vi "get_all_refr_pol_corrections.vi"(8 "Error In":errorcluster, 10 "Sample":string, 11 "File Path":path) -> (0 "Error Out":errorcluster)   [LabVIEW 2019]
panel:
  out "Progress":u8(slide) scale=0.0..100.0
  # "Refration and Polarization Correction"
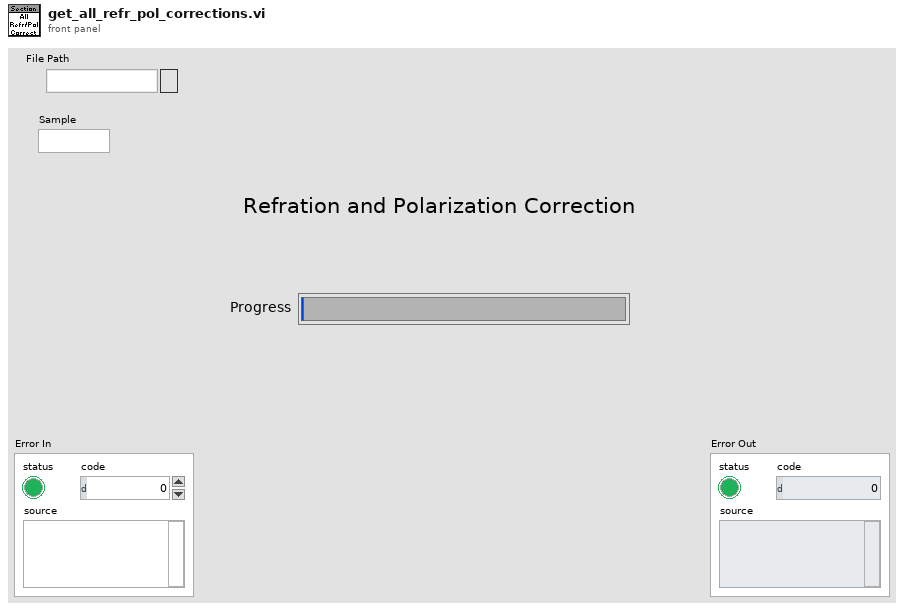
[diagram p1: front panel]
types:
  T1 = cluster{"xi":dbl, "phiin":dbl, "expected extinction angle":dbl, "a":dbl, "b":dbl, "m1":dbl, "m2":dbl, "m3":dbl, "D":dbl}
  T2 = typedef "sample_results_cluster_typedef.ctl" = cluster{"File Path":string, "Sample":string, "Threshold":dbl, "Parameters":T3, "Writeable Parameters":T4, "Gain Results":T5[]}
  T3 = typedef "parameters_cluster_typedef.ctl" = cluster{"m1":dbl, "m2":dbl, "m3":dbl, "c":dbl, "D":dbl, "Beta":dbl, "center x":dbl, "center y":dbl}
  T4 = typedef "writeable_section_parameters_cluster_typedef.ctl" = cluster{"Section":string, "Method":i32, "Edge Mode":i32, "Grid Constant":i32, "Manual Sequence":i32, "ROI Size":i32, "Min Grain Size":dbl, "Comments":string, "File Path":string}
  T5 = typedef "grain_results_cluster_typedef.ctl" = cluster{"Grain Number":i32, "xi":dbl[], "phiin":dbl[], "Intensity":dbl[][], "Best Fit Intensity":dbl[][], "Best Fit Parameters":dbl[][], "Polarizer 1 Angle":dbl[][], "Polarizer 2 Angle":dbl[][], "Best Extinction Angle":dbl[], "Best Extinction Angle Corrected":dbl[], "Thetac":dbl, "Phic":dbl, "ROI":cluster{"Global Rectangle":i32[], "Contours":cluster{"Contour Type":u32, "ROI Type":u32, "Points":i32[]}[]}, "a":dbl, "b":dbl, "sequences available":dbl, "sequences used":dbl, "Contrast":dbl[], "Rsq":dbl}
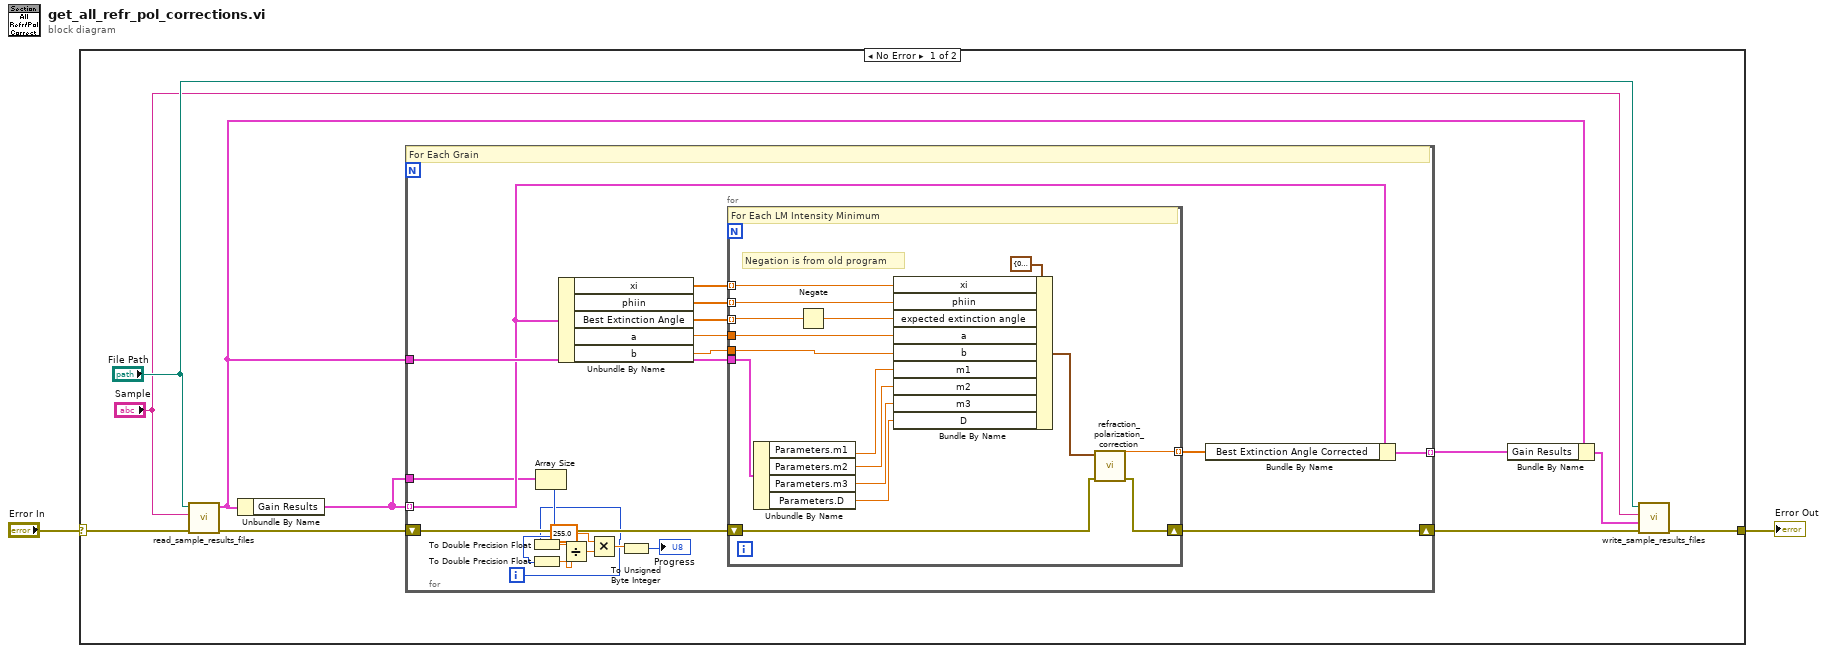
[diagram p0: block diagram]
diagram:
  n1 = case shown="No Error" "Error In" {
    selector: "Error In" -> [w12 w49]
    tunnel: [w7 w49] -> w1
    frame No Error {
      n2 = call "read_sample_results_files.vi"("Error In"=w12, "Sample"="Sample", "File Path"="File Path") -> ("Error Out"=w11:errorcluster, "Sample Results"=w10:T2)  [unwired: 7 in]
      n3 = Unbundle By Name(w10) -> ("Gain Results"=w3:T5[])
      n4 = for {
        tunnel: w3 -> [w26] mode=indexing
        tunnel: w10 -> [w29]
        shift-right: [w27] -> w8
        shift-left: w11 -> [w28]
        tunnel: [w25] -> w9 mode=indexing
        tunnel: w3 -> [w17]
        i -> [w18]
        # "For Each Grain"
        n5 = To Double Precision Float(number=w18) -> (double precision float=w20:dbl)
        n6 = Array Size(array=w17) -> (size(s)=w21:i32)
        n7 = To Double Precision Float(number=w21) -> (double precision float=w16:dbl)
        n8 = Unbundle By Name(w26) -> ("xi"=w32:dbl[], "phiin"=w31:dbl[], "Best Extinction Angle"=w30:dbl[], "a"=w14:dbl, "b"=w13:dbl)
        n9 = Divide(x=w20, y=w16) -> (x/y=w22:dbl)
        n10 = Multiply(x=255.0, y=w22) -> (x*y=w23:dbl)
        n11 = To Unsigned Byte Integer(number=w23) -> (unsigned 8bit integer=→"Progress":u8)
        n12 = for {
          tunnel: w32 -> [w46] mode=indexing
          tunnel: w31 -> [w45] mode=indexing
          tunnel: w30 -> [w37] mode=indexing
          tunnel: w29 -> [w44]
          shift-right: [w38] -> w27
          shift-left: w28 -> [w39]
          tunnel: [w35] -> w15 mode=indexing
          tunnel: w14 -> [w34]
          tunnel: w13 -> [w33]
          # "Negation is from old program"
          # "For Each LM Intensity Minimum"
          n13 = Unbundle By Name(w44) -> ("Parameters.m1"=w43:dbl, "Parameters.m2"=w42:dbl, "Parameters.m3"=w41:dbl, "Parameters.D"=w40:dbl)
          n14 = Negate(x=w37) -> (-x=w36:dbl)
          n15 = Bundle By Name(cluster=T1 {"xi"=0.0, "phiin"=0.0, "expected extinction angle"=0.0, "a"=0.0, "b"=0.0, "m1"=0.0, "m2"=0.0, "m3"=0.0, "D"=0.0} ("Refraction Polarization Correction Input"), "xi"=w46, "phiin"=w45, "expected extinction angle"=w36, "a"=w34, "b"=w33, "m1"=w43, "m2"=w42, "m3"=w41, "D"=w40) -> (w47:T1)
          n16 = call "refraction_polarization_correction.vi"("Error In"=w39, "Refraction Polarization Correction Input"=w47) -> ("Error Out"=w38:errorcluster, "corrected angle"=w35:dbl)  [unwired: 8 in]
        }
        n17 = Bundle By Name(cluster=w26, "Best Extinction Angle Corrected"=w15) -> (w25:T5)
      }
      n18 = Bundle By Name(cluster=w10, "Gain Results"=w9) -> (w6:T2)
      n19 = call "write_sample_results_files.vi"("Error In"=w8, "Sample Results"=w6, "Sample"="Sample", "File Path"="File Path") -> ("Error Out"=w7:errorcluster)  [unwired: 7 in]
    }
    frame Error {
    }
  }
  "Error Out" <- w1
